vi "IniFileArray.vi"(8 "ErrorArray In":errorcluster[](array[cluster]), 10 "Relative Path to Plugins":path=path "") -> (0 "ErrorArray Out":errorcluster[](array[cluster]), 2 "INIFilePaths":path[](array[path]))   [LabVIEW 2014, in "Ini_lib.lvlib"]
uses:
  Ini_lib.lvlib
  <userlib>/NIST/NISTErrorLib/NISTErrorLib.lvlib
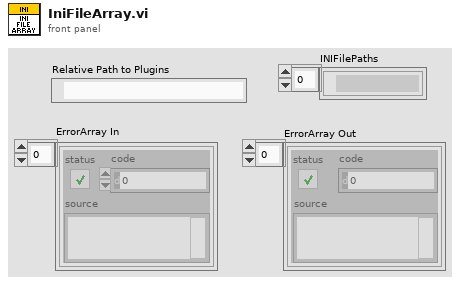
[diagram p1: front panel]
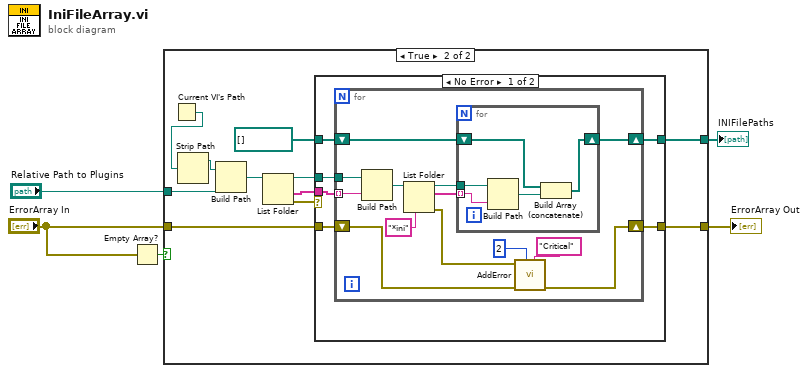
[diagram p0: block diagram]
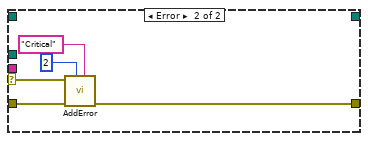
[diagram p3: hidden frame]
diagram:
  n1 = Empty Array?(array="ErrorArray In") -> (empty?=w5:bool)
  n2 = case shown="True" w5 {
    tunnel: "ErrorArray In" -> [w6 w14]
    tunnel: "Relative Path to Plugins" -> [_ w16]
    tunnel: [w6 w13] -> w2
    tunnel: [_ w9] -> w1
    frame False {
    }
    frame True {
      n3 = Current VI's Path() -> (path=w7:path)
      n4 = Strip Path(path=w7) -> (stripped path=w8:path)  [unwired: 1 out]
      n5 = Build Path(base path=w8, name or relative path=w16) -> (appended path=w17:path)
      n6 = List Folder(path=w17) -> (path out=w10:path, folder names=w11:string[], error out=w15:errorcluster)  [unwired: 3 in, 1 out]
      n7 = case shown="No Error" w15 {
        selector: w15 -> [_ w45]
        tunnel: w14 -> [w20 w46]
        tunnel: [w19 w42] -> w13
        tunnel: path[] [] ("EvtINIFilePaths 2") -> [w23 _]
        tunnel: w11 -> [w22 _]
        tunnel: w10 -> [w21 _]
        tunnel: [w18 _] -> w9
        frame No Error {
          n8 = for {
            shift-right: [w29] -> w18
            shift-left: w23 -> [w30]
            tunnel: w22 -> [w32] mode=indexing
            tunnel: w21 -> [w33]
            shift-right: [w27] -> w19
            shift-left: w20 -> [w28]
            n9 = Build Path(base path=w33, name or relative path=w32) -> (appended path=w35:path)
            n10 = List Folder(path=w35, pattern="*ini") -> (path out=w31:path, filenames=w34:string[], error out=w24:errorcluster)  [unwired: 2 in, 1 out]
            n11 = for {
              tunnel: w34 -> [w39] mode=indexing
              tunnel: w31 -> [w40]
              shift-right: [w38] -> w29
              shift-left: w30 -> [w37]
              n12 = Build Path(base path=w40, name or relative path=w39) -> (appended path=w41:path)
              n13 = Build Array (concatenate)(w37, w41) -> (w38:path[])
            }
            n14 = call <userlib>:"AddError.vi"("Severity"="Critical", "Priority"=u8 2, "ErrorArray"=w28, "error in (no error)"=w24) -> ("ErrorArray"=w27:errorcluster[])  [unwired: 6 in, 1 out]
          }
        }
        frame Error {
          n15 = call <userlib>:"AddError.vi"("Severity"="Critical", "Priority"=u8 2, "ErrorArray"=w46, "error in (no error)"=w45) -> ("ErrorArray"=w42:errorcluster[])  [unwired: 6 in, 1 out]
        }
      }
    }
  }
  "ErrorArray Out" <- w2
  "INIFilePaths" <- w1
